vi "UTF-16 Byte Swap.vi"(1 "String in":string) -> (0 "String out":string)   [LabVIEW 2020, in "G-Unicode.lvlib"]
doc: "Swaps the byte order of a UTF-16 encoded string."
uses:
  G-Unicode.lvlib
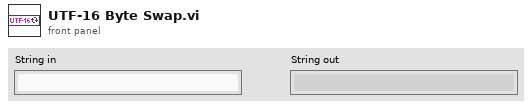
[diagram p1: front panel]
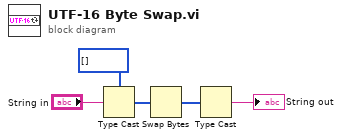
[diagram p0: block diagram]
diagram:
  n1 = Type Cast(type=u16[] [] ("unsigned byte array"), x="String in") -> (*(type *) &x=w4:u16[])
  n2 = Swap Bytes(anything=w4) -> (byte swapped=w3:u16[])
  n3 = Type Cast(x=w3) -> (*(type *) &x=→"String out":string)  [unwired: 1 in]
